vi "test Import Same Module Same Configuration.vi"(8 "error in (no error)":errorcluster, 11 "TestCase in":refnum<class "SLSC Switch Import Unit Tests.lvclass">) -> (0 "error out":errorcluster, 3 "TestCase out":refnum<class "SLSC Switch Import Unit Tests.lvclass">)   [LabVIEW 2017, in "SLSC Switch Import Unit Tests.lvclass"]
uses:
  SLSC Switch Import Unit Tests.lvclass
  Shared/Endpoint Configuration Cluster.ctl
  Shared/Endpoint Configuration Enum.ctl
  SLSC Switch Import Unit Tests.lvclass/SLSC Switch Import Unit Tests.ctl
  <vilib>/addons/_JKI Toolkits/VI Tester/TestCase.llb/TestCase.lvclass
  <vilib>/NI/NI VeriStand Custom Device Import and Export Tool/ImportExport.lvlib
  Scripting/SLSC Switch Scripting.lvlib
  Shared/SLSC Switch Shared.lvlib
  C:/Program Files (x86)/National Instruments/LabVIEW 2017/vi.lib/addons/_JKI Toolkits/VI Tester/TestCase.llb/TestCase.lvclass
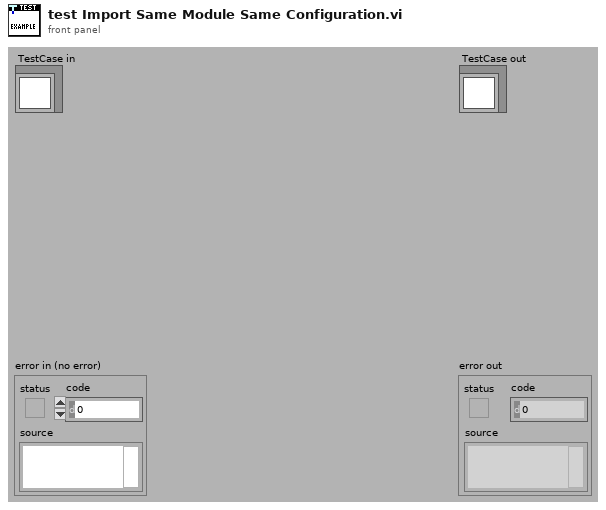
[diagram p1: front panel]
types:
  T1 = cluster{"Ignore Properties":string[], "Ignore Top Level Name":bool}
  T2 = typedef "SLSC Switch Shared.lvlib/Endpoint Configuration Cluster.ctl" = cluster{"Endpoint":string, "Configuration":T3}
  T3 = typedef "SLSC Switch Shared.lvlib/Endpoint Configuration Enum.ctl" = enum16{"Load", "Source", "Configuration"}
  T4 = typedef "Custom Device API.lvlib/Custom Device Item Ref.ctl" = u64
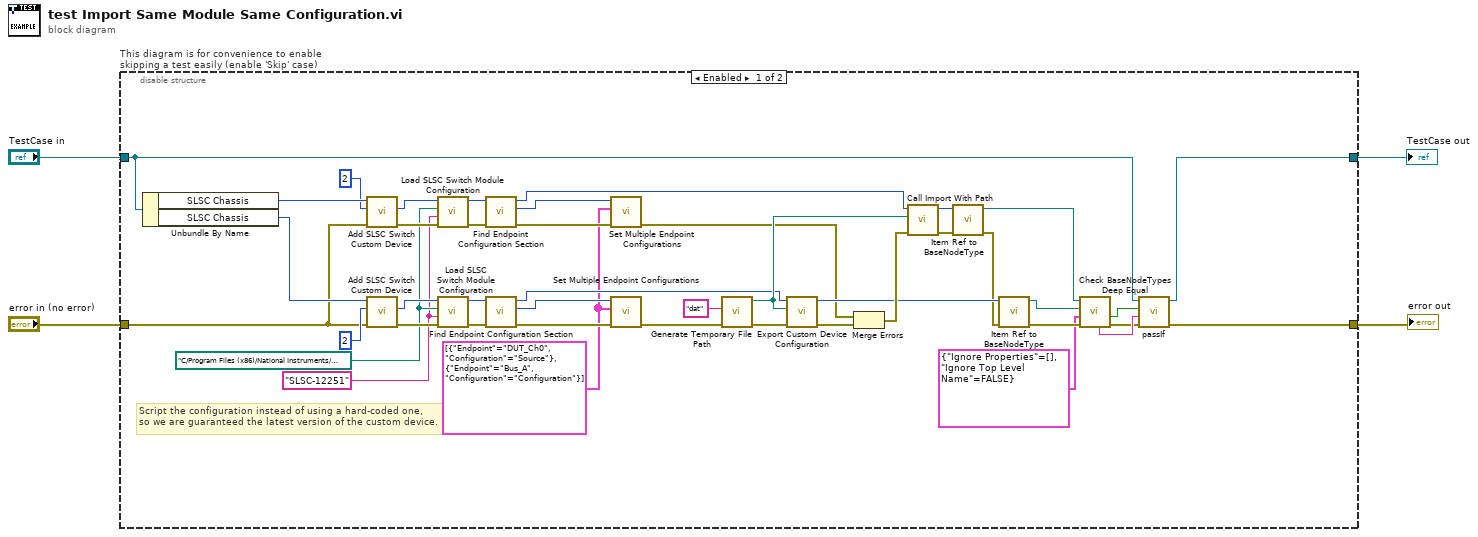
[diagram p0: block diagram]
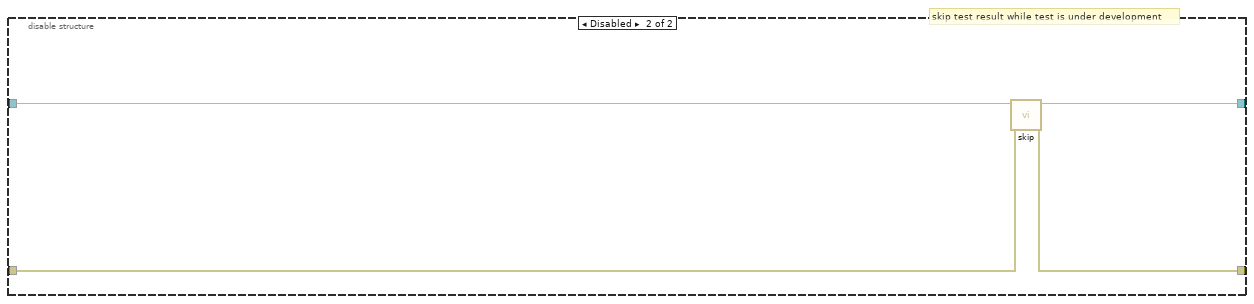
[diagram p2: hidden frame]
diagram:
  n1 = disable-structure "This diagram is for convenience to enable skipping a test easily (enable 'Skip' case)" shown="Enabled" {
    disable-tunnel: "TestCase in" -> [w34 w51]
    disable-tunnel: [w6 w49] -> w1
    disable-tunnel: [w5 w50] -> w3
    disable-tunnel: "error in (no error)" -> [w28 w48]
    frame Enabled {
      w10 = T2[] [{"Endpoint"="DUT_Ch0", "Configuration"=enum."Source"}, {"Endpoint"="Bus_A", "Configuration"=enum."Configuration"}] ("endpoint configurations")
      w14 = path "C:/Program Files (x86)/National Instruments/Shared/NI-SLSC Switch/Modules/SLSC-12251-switches.json" ("switches json file")
      w13 = "SLSC-12251" ("product name")
      # "Script the configuration instead of using a hard-coded one,\nso we are guaranteed the latest version of the custom device."
      n2 = Unbundle By Name(w34) -> ("SLSC Chassis"=w29:u64, "SLSC Chassis"=w47:u64)
      n3 = call "Add SLSC Switch Custom Device.vi"("error in"=w28, "slot number"=u32 2, "slsc chassis in"=w29) -> ("error out"=w16:errorcluster, "slsc switch custom device"=w12:T4)  [unwired: 6 in, 1 out]
      n4 = call "Add SLSC Switch Custom Device.vi"("error in"=w28, "slot number"=u32 2, "slsc chassis in"=w47) -> ("error out"=w27:errorcluster, "slsc switch custom device"=w25:T4)  [unwired: 6 in, 1 out]
      n5 = call "Load SLSC Switch Module Configuration.vi"("error in"=w16, "product name"=w13, "switches json file"=w14, "slsc switch custom device in"=w12) -> ("error out"=w15:errorcluster, "slsc switch custom device out"=w17:T4)  [unwired: 6 in]
      n6 = call "Load SLSC Switch Module Configuration.vi"("error in"=w27, "product name"=w13, "switches json file"=w14, "slsc switch custom device in"=w25) -> ("error out"=w26:errorcluster, "slsc switch custom device out"=w23:T4)  [unwired: 6 in]
      n7 = call "Find Endpoint Configuration Section.vi"("error in"=w15, "slsc switch custom device in"=w17) -> ("error out"=w11:errorcluster, "endpoint configuration"=w9:T4, "slsc switch custom device out"=w8:T4)  [unwired: 7 in]
      n8 = call "Find Endpoint Configuration Section.vi"("error in"=w26, "slsc switch custom device in"=w23) -> ("error out"=w24:errorcluster, "endpoint configuration"=w21:T4, "slsc switch custom device out"=w20:T4)  [unwired: 7 in]
      n9 = call "Set Multiple Endpoint Configurations.vi"("error in"=w11, "endpoint configurations"=w10, "endpoint configuration in"=w9) -> ("error out"=w7:errorcluster)  [unwired: 7 in, 1 out]
      n10 = call "Set Multiple Endpoint Configurations.vi"("error in"=w24, "endpoint configurations"=w10, "endpoint configuration in"=w21) -> ("error out"=w22:errorcluster)  [unwired: 7 in, 1 out]
      n11 = call <vilib>:"Generate Temporary File Path.vi"("error in (no error)"=w22, "Temporary File Extension (tmp)"="dat") -> ("error out"=w44:errorcluster, "Unique Temporary File Path"=w41:path)  [unwired: 8 in]
      n12 = call <vilib>:"Export Custom Device Configuration.vi"("error in (no error)"=w44, "Path"=w41, "ID"=w20) -> ("error out"=w43:errorcluster, "ID out"=w39:u64)  [unwired: 7 in]
      n13 = Merge Errors(w7, w43) -> (w42:errorcluster)
      n14 = call "Call Import With Path.vi"("error in (no error)"=w42, "Path"=w41, "Node Ptr"=w8) -> ("error out"=w38:errorcluster, "Node Ptr out"=w40:u64)  [unwired: 7 in]
      n15 = call "Item Ref to BaseNodeType.vi"("error in (no error)"=w38, "Item Ref"=w40) -> ("error out"=w37:errorcluster, "BaseNodeType"=w31:refnum<k24>)  [unwired: 8 in]
      n16 = call "Item Ref to BaseNodeType.vi"("error in (no error)"=w37, "Item Ref"=w39) -> ("error out"=w36:errorcluster, "BaseNodeType"=w35:refnum<k24>)  [unwired: 8 in]
      n17 = call "Check BaseNodeTypes Deep Equal.vi"("error in (no error)"=w36, "Settings"=T1 {"Ignore Properties"=[], "Ignore Top Level Name"=FALSE}, "BaseNodeType 2"=w35, "BaseNodeType 1"=w31) -> ("error out"=w30:errorcluster, "Equal?"=w33:bool, "Inequality context"=w32:string)  [unwired: 3 in, 2 out]
      n18 = call-dynamic "passIf.vi"("error in (no error)"=w30, "message (\"\")"=w32, "pass"=w33, "TestCase in"=w34) -> ("error out"=w5:errorcluster, "TestCase out"=w6:refnum<class "SLSC Switch Import Unit Tests.lvclass">)  [unwired: 6 in]
    }
    frame Disabled {
      # "skip test result while test is under development"
      n19 = call <vilib>:"skip.vi"("error in (no error)"=w48, "TestCase in"=w51) -> ("error out"=w50:errorcluster, "TestCase out"=w49:refnum<class "SLSC Switch Import Unit Tests.lvclass">)  [unwired: 8 in]
    }
  }
  "error out" <- w3
  "TestCase out" <- w1
